vi "RT Control FGV.vi"(7 "Enum":enum16{"Read", "Write"}(ring), 11 "RT Ctrl":cluster{"RT IP":string, "RT Connect":bool}={"RT IP"="localhost", "RT Connect"=FALSE}) -> (3 "RT Ctrl out":cluster{"RT IP":string, "RT Connect":bool})   [LabVIEW 2022 SP3]
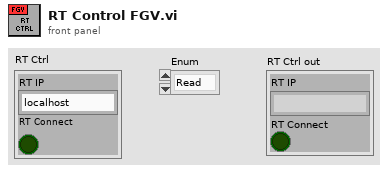
[diagram p1: front panel]
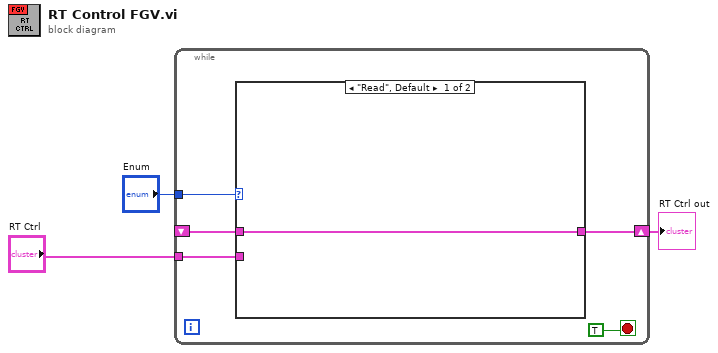
[diagram p0: block diagram]
diagram:
  n1 = while {
    tunnel: "Enum" -> [w8]
    tunnel: "RT Ctrl" -> [w6]
    shift-right: [w5] -> w1
    shift-left: _ -> [w4]
    stop <- TRUE stop-if-true
    n2 = case shown="\"Read\", Default" w8 {
      tunnel: w6 -> [_ w10]
      tunnel: [w9 w10] -> w5
      tunnel: w4 -> [w9 _]
      frame "Read", Default {
      }
      frame "Write" {
      }
    }
  }
  "RT Ctrl out" <- w1
